vi "Convert s_Float to ms_I32.vi"(1 "Seconds IN (Float)":dbl) -> (0 "milliseconds OUT (I32)":i32)   [LabVIEW 2017]
doc: "SciScan 1.2 160622\nThis VI converts a seconds input (floating point) to a millisecond(I32) output.\nThe VI execution is configured to run as 'inline code', with re-entrant execution. The reason for this is considering its small size and the relative overhead that a function call would incur."
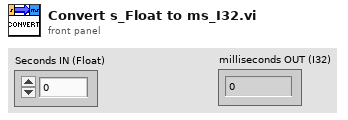
[diagram p1: front panel]
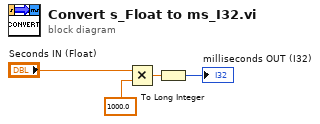
[diagram p0: block diagram]
diagram:
  n1 = Multiply(x="Seconds IN (Float)", y=1000.0) -> (x*y=w4:dbl)
  n2 = To Long Integer(number=w4) -> (32bit integer=→"milliseconds OUT (I32)":i32)
